vi "Mercury Open.vi"(8 "Error In":errorcluster, 11 "VISA resource name":refnum<visa-resource-name>) -> (0 "Error Out":errorcluster, 3 "VISA resource name out":refnum<visa-resource-name>)   [LabVIEW 2019]
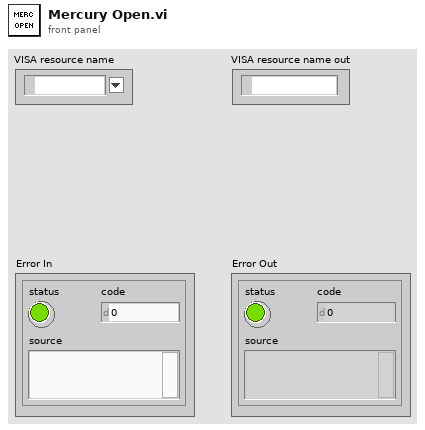
[diagram p1: front panel]
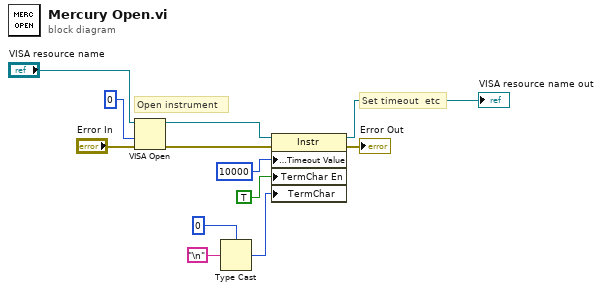
[diagram p0: block diagram]
diagram:
  # "Set timeout  etc"
  # "Open instrument"
  n1 = VISA Open(access mode=u32 0, error in (no error)="Error In", VISA resource name="VISA resource name") -> (VISA resource name=w4:refnum<visa-resource-name>, error out=w3:errorcluster)  [unwired: 2 out]
  n2 = Type Cast(type=u8 0 ("Message Based Settings:Termination Character"), x="\n") -> (*(type *) &x=w9:u8)
  n3 = property on="Property Node" class="Instr"(reference=w4, error in=w3, "General Settings:Timeout Value"=u32 10000, "TermChar En"=TRUE ("Message Based Settings:Termination Character Enable"), "TermChar"=w9) -> (reference out=→"VISA resource name out":refnum<visa-resource-name>, error out=→"Error Out":errorcluster)
